vi "Collect_Coordinates(X,Y)_in_Array.vi"(2 "Initial Index \nfor Replacement":i32, 3 "[IN] Array for \nCollecting \nCoord (X,Y)":dbl[](array[numeric]), 4 "Y":dbl, 5 "X":dbl) -> (0 "Finish\nIndex":i32, 1 "[OUT] Array\nfor collecting":dbl[](array[numeric]))   [LabVIEW 2017]
doc: "Saves coordinates (X,Y) in the array"
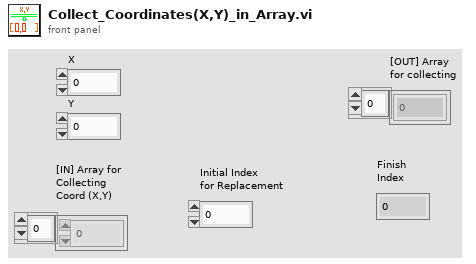
[diagram p1: front panel]
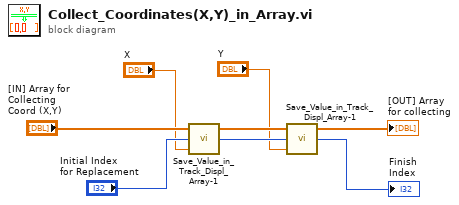
[diagram p0: block diagram]
diagram:
  n1 = call "Save_Value_in_Track_Displ_Array-1.vi"("[IN] Value"="X", "[IN] Index"="Initial Index \nfor Replacement", "[IN] Empty tracks\nfor points saving"="[IN] Array for \nCollecting \nCoord (X,Y)") -> ("[OUT] Index ++"=w3:i32, "[OUT Track with saved value"=w4:dbl[])  [unwired: 1 in]
  n2 = call "Save_Value_in_Track_Displ_Array-1.vi"("[IN] Value"="Y", "[IN] Index"=w3, "[IN] Empty tracks\nfor points saving"=w4) -> ("[OUT] Index ++"=→"Finish\nIndex":i32, "[OUT Track with saved value"=→"[OUT] Array\nfor collecting":dbl[])  [unwired: 1 in]
